vi "Autonomous Independent.vi"() -> ()   [LabVIEW 2018]
doc: "This VI is called when autonomous begins, and will automatically be terminated when autonomous ends. You can carry out timed or sensor driven robot movement independently without needing to return to the caller."
uses:
  <vilib>/Analysis/baseanly.llb/Mean (DBL).vi
  <vilib>/Rock Robotics/WPI/Utilities/WPI_GetSetVariantRefNum.vi
  <vilib>/Rock Robotics/Network Tables/NT Read Number.vi
  <vilib>/Rock Robotics/Network Tables/NT Write Numeric Array.vi
  <vilib>/Rock Robotics/Network Tables/NT Write String.vi
  Robot Global Data.vi
  <vilib>/Rock Robotics/WPI/RobotDrive/WPI_RobotDriveArcadeDrive_Standard(NoSaturation).vi
  <vilib>/Rock Robotics/Network Tables/NT Write Number.vi
  <vilib>/Analysis/NI_AALBase.lvlib
panel:
  in  "Array of robot movements":T1(array[cluster])=[{"X Joystick Value"=0.39393939393939403, "Y Joystick Value"=0.0, "Delay (sec)"=1.0, "Movement Name"="turn"}, {"X Joystick Value"=-0.3737373737373737, "Y Joystick Value"=0.0, "Delay (sec)"=1.0, "Movement Name"="turn back"}] {"Y Joystick Value" scale=1.0..-1.0; "X Joystick Value" scale=-1.0..1.0}
  out "Current Movement, for debugging":T2 {"Y Joystick Value" scale=1.0..-1.0; "X Joystick Value" scale=-1.0..1.0}
  # "Be sure to right-click and choose Data Operations>>Make Current Value default if you want to save the array values with the VI"
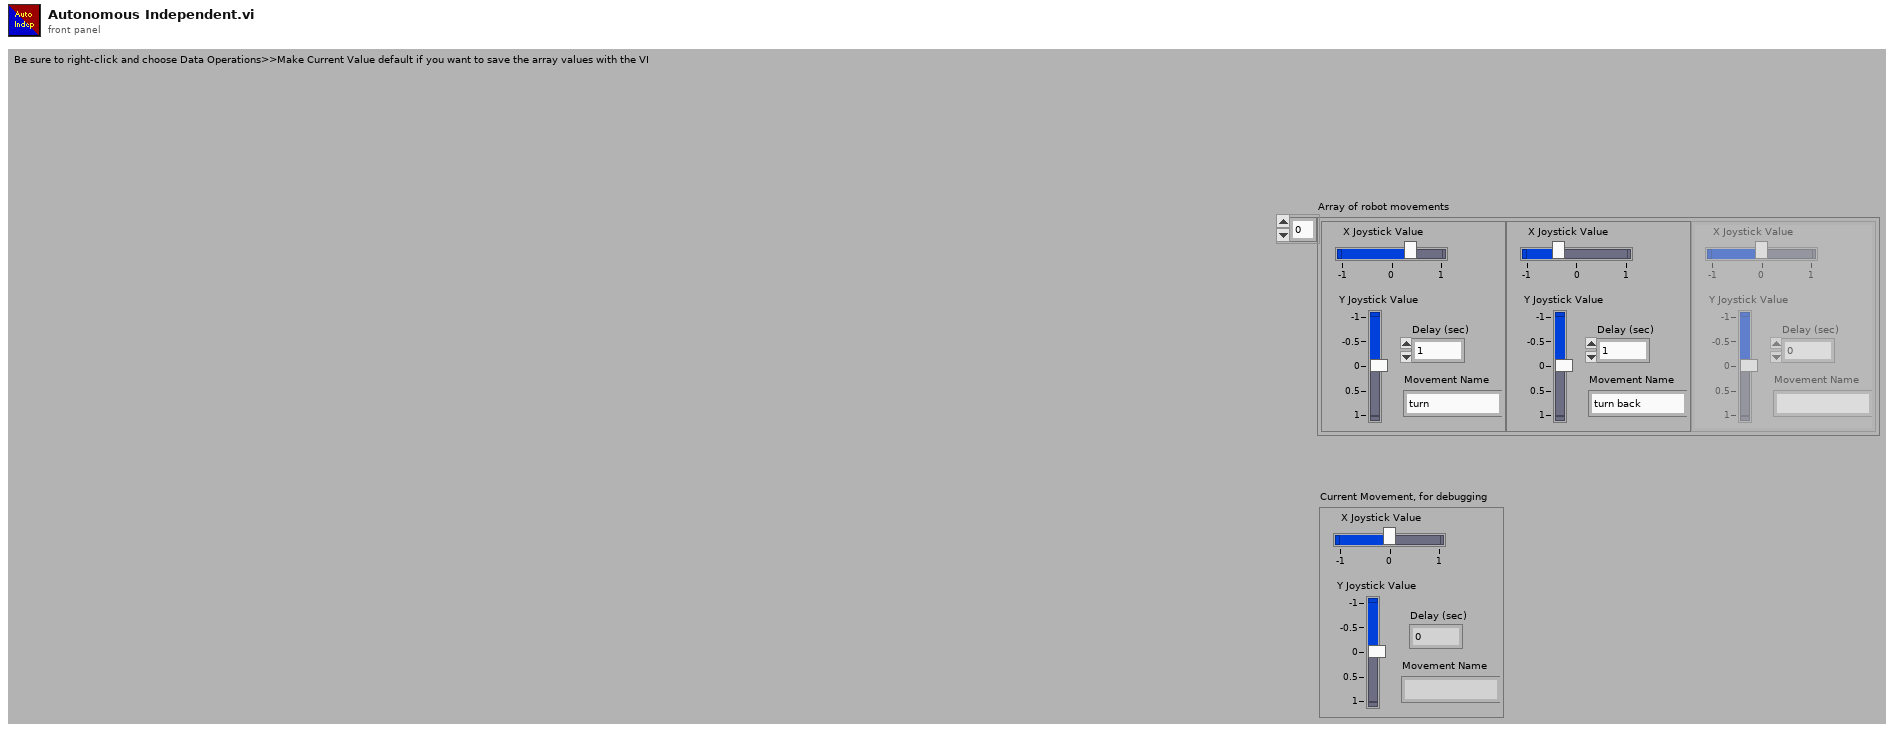
[diagram p1: front panel]
types:
  T1 = cluster{"X Joystick Value":dbl, "Y Joystick Value":dbl, "Delay (sec)":dbl, "Movement Name":string}[]
  T2 = cluster{"X Joystick Value":dbl, "Y Joystick Value":dbl, "Delay (sec)":dbl, "Movement Name":string}
  T3 = typedef "WPI_JoystickDevRef.ctl" = cluster{"Device":T4}
  T4 = typedef "WPI_JoystickDeviceEnum.ctl" = enum16{"USB 0", "USB 1", "USB 2", "USB 3", "USB 4", "USB 5"}
  T5 = typedef "WPI_RobotDriveDevRef.ctl" = cluster{"DevStatus":errorcluster, "Motors[]":T6[], "Square Inputs":bool, "Max Output":dbl}
  T6 = typedef "WPI_MotorControlDeviceRef.ctl" = cluster{"DeviceStatus":errorcluster, "Type":T7, "PWM":cluster{"PWM Channel":T8, "DeadBand":T9}, "CAN":cluster{"Device Number":u8, "SetOutput VI Ref":variant, "GetOutput VI Ref":variant, "Enable VI Ref":variant, "Disable VI Ref":variant, "Data":variant}, "Invert":bool, "DIO PWM":cluster{"PWM \"Enable\" Channel":T8, "DIOChannel":T10, "PWM Rate":dbl}}
  T7 = typedef "WPI_MotorControlType.ctl" = enum16{"PWM", "CAN", "DIO PWM"}
  T8 = typedef "FPGA_DIOPWMChannel.ctl" = enum8{"PWM 0", "PWM 1", "PWM 2", "PWM 3", "PWM 4", "PWM 5", "PWM 6", "PWM 7", "PWM 8", "PWM 9", "PWM MXP 0", "PWM MXP 1", "PWM MXP 2", "PWM MXP 3", "PWM MXP 4", "PWM MXP 5", "PWM MXP 6", "PWM MXP 7", "PWM MXP 8", "PWM MXP 9", "Invalid"}
  T9 = typedef "WPI_PWMDeadband.ctl" = cluster{"Name":string, "maxPositivePwm":i32, "minPositivePwm":i32, "centerPwm":i32, "maxNegativePwm":i32, "minNegativePwm":i32, "angularRange":u16}
  T10 = typedef "FPGA_DIOChannel.ctl" = enum8{"DIO 0", "DIO 1", "DIO 2", "DIO 3", "DIO 4", "DIO 5", "DIO 6", "DIO 7", "DIO 8", "DIO 9", "DIO MXP 0", "DIO MXP 1", "DIO MXP 2", "DIO MXP 3", "DIO MXP 4", "DIO MXP 5", "DIO MXP 6", "DIO MXP 7", "DIO MXP 8", "DIO MXP 9", "DIO MXP 10", "DIO MXP 11", "DIO MXP 12", "DIO MXP 13", "DIO MXP 14", "DIO MXP 15", "SPI Port CS1", "SPI Port CS2", "SPI Port CS3", "SPI Port MISO", "SPI Port MOSI", "Invalid"}
  T11 = typedef "WPI_AnalogChannelDevRef.ctl" = cluster{"DevStatus":errorcluster, "Analog Channel":T12}
  T12 = typedef "FPGA_AIChannel.ctl" = enum8{"AI 0", "AI 1", "AI 2", "AI 3", "AI MXP 0", "AI MXP 1", "AI MXP 2", "AI MXP 3", "Invalid"}
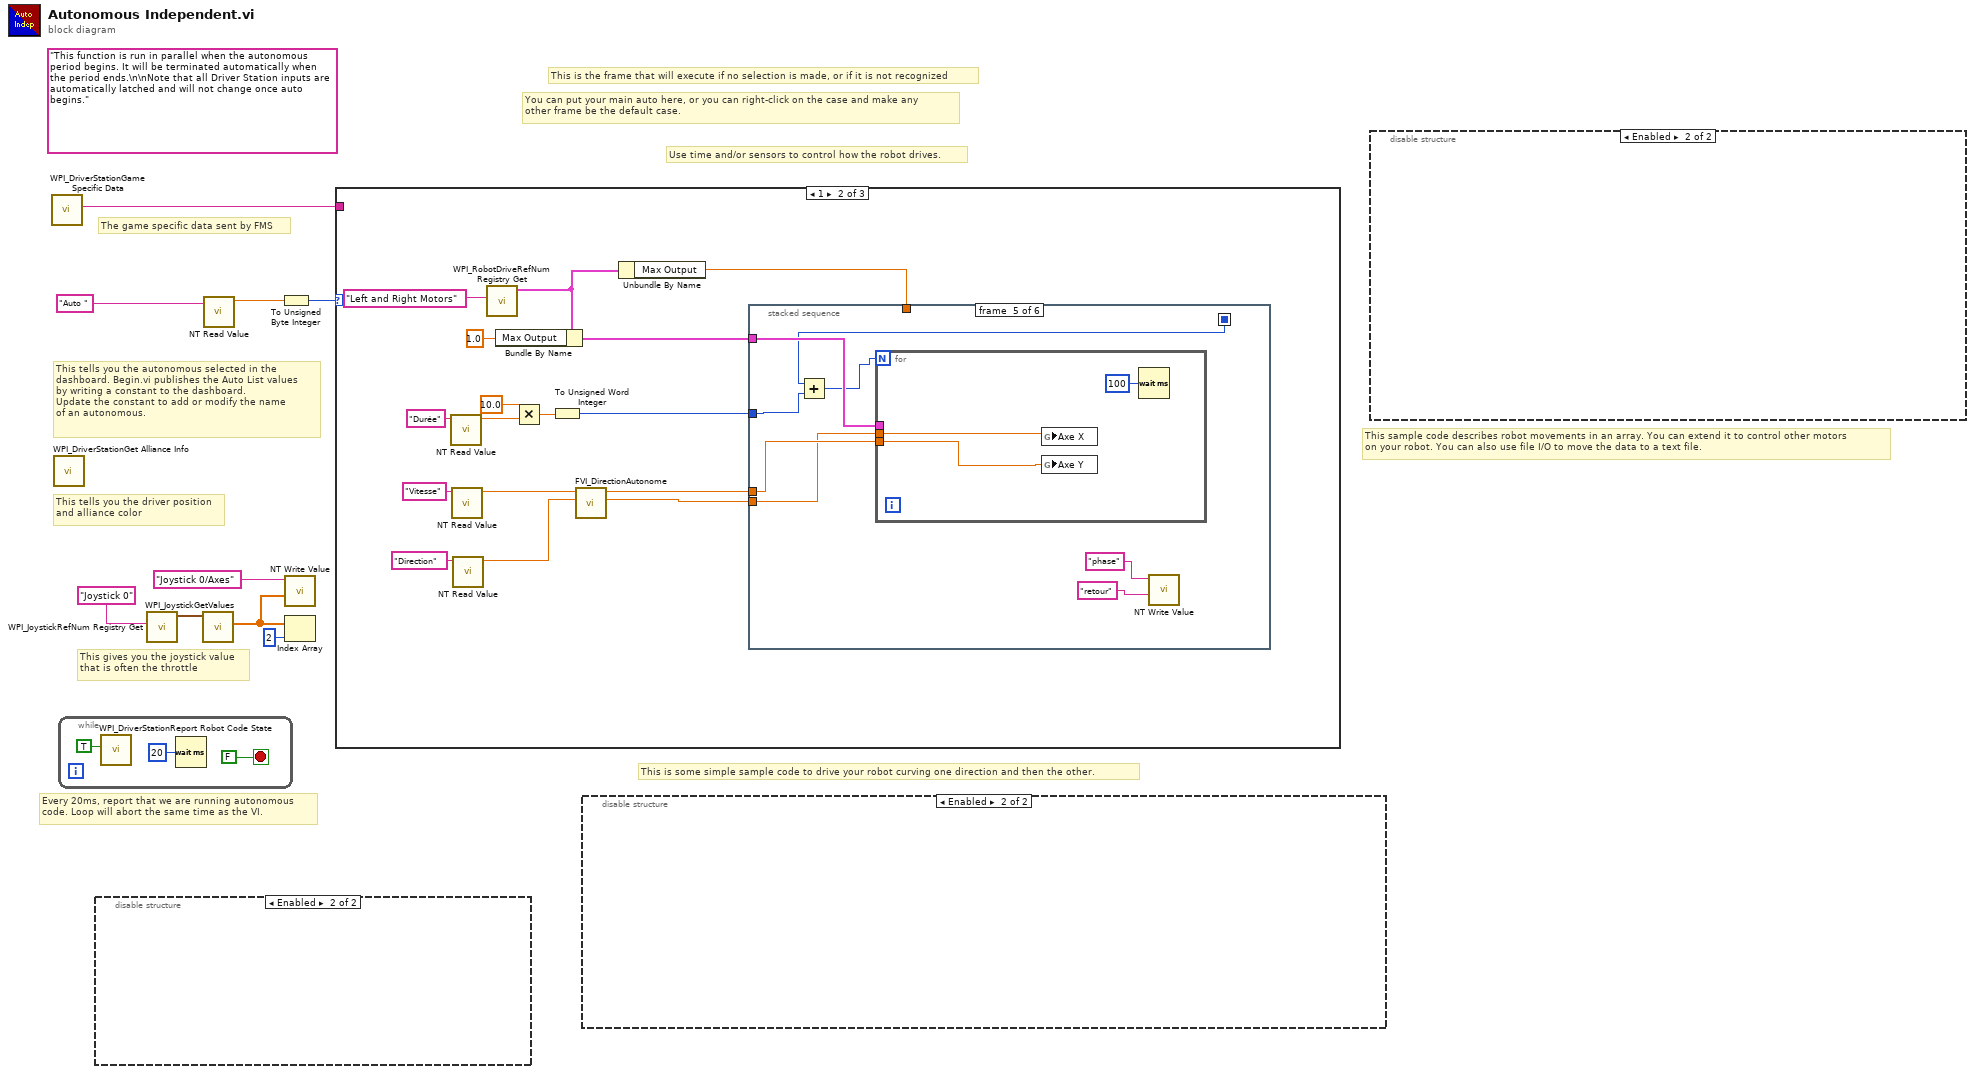
[diagram p0: block diagram]
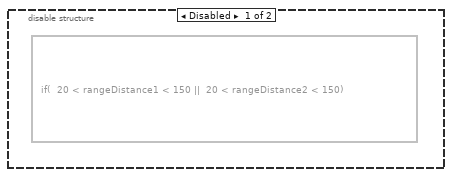
[diagram p2: hidden frame]
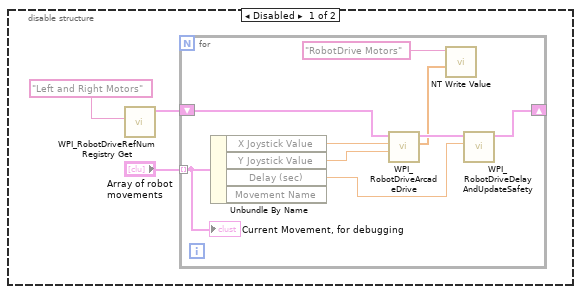
[diagram p3: hidden frame]
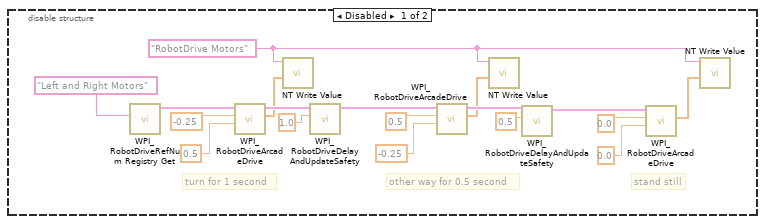
[diagram p4: hidden frame]
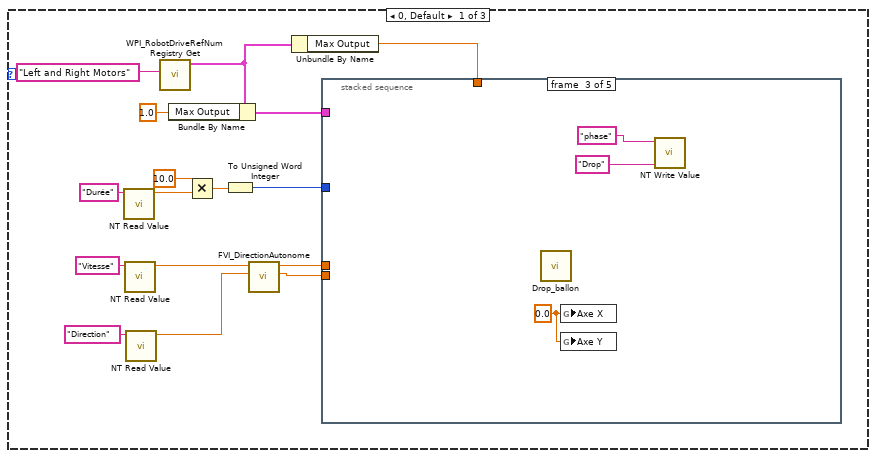
[diagram p5: hidden frame]
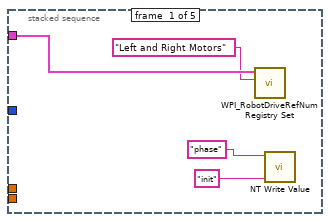
[diagram p6: hidden frame]
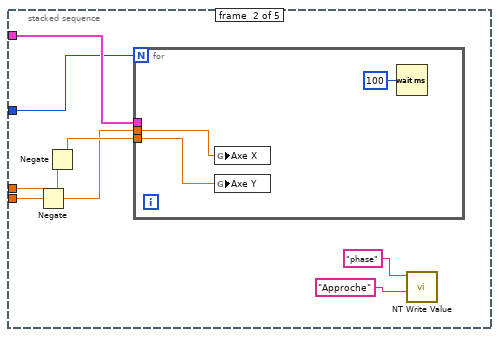
[diagram p7: hidden frame]
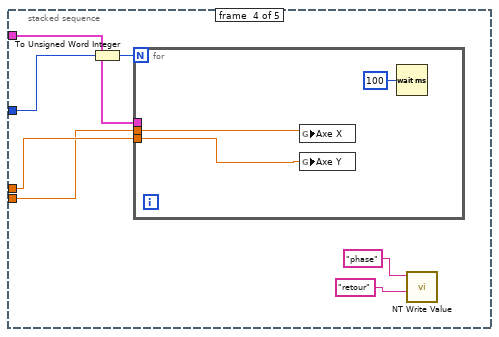
[diagram p8: hidden frame]
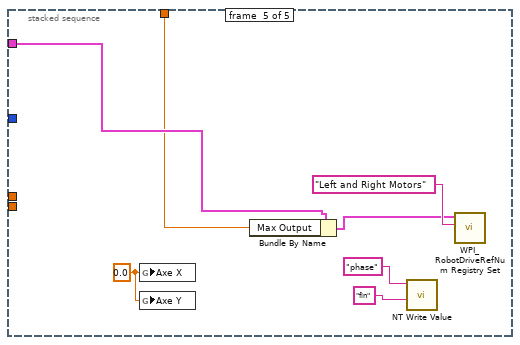
[diagram p9: hidden frame]
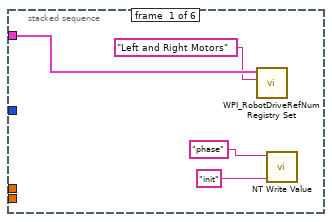
[diagram p10: hidden frame]
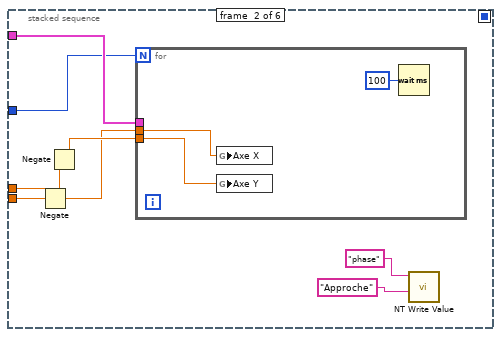
[diagram p11: hidden frame]
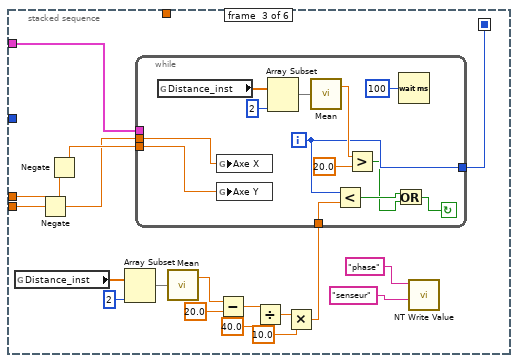
[diagram p12: hidden frame]
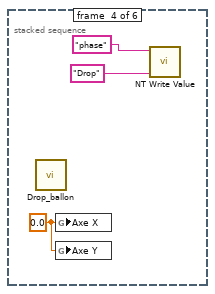
[diagram p13: hidden frame]
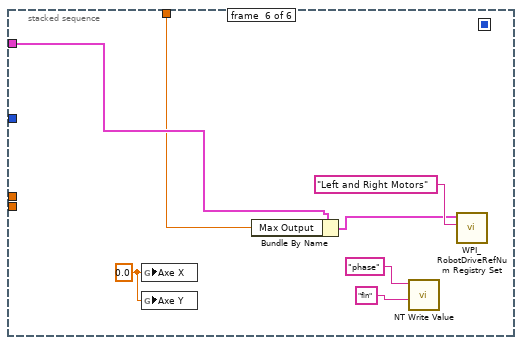
[diagram p14: hidden frame]
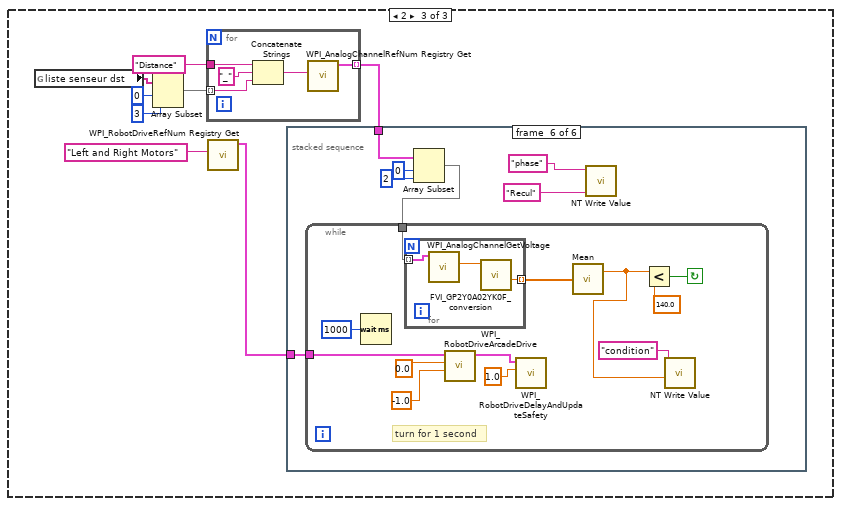
[diagram p15: hidden frame]
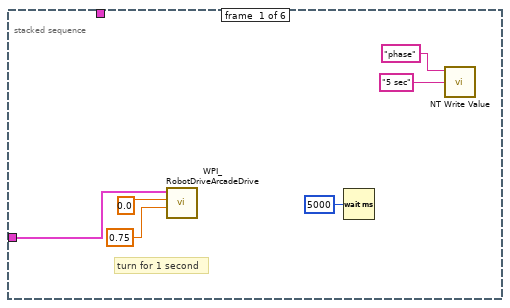
[diagram p16: hidden frame]
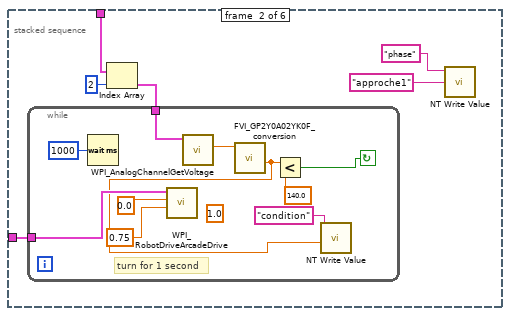
[diagram p17: hidden frame]
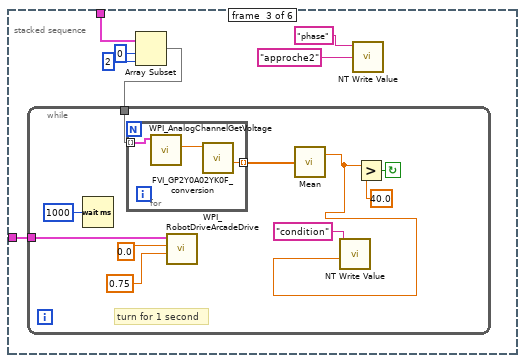
[diagram p18: hidden frame]
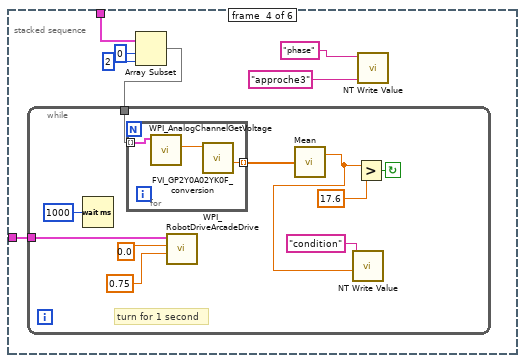
[diagram p19: hidden frame]
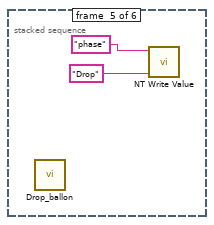
[diagram p20: hidden frame]
diagram:
  (unwired) "This function is run in parallel when the autonomous period begins. It will be terminated automatically when the period ends.\n\nNote that all Driver Station inputs are automatically latched and will not change once auto begins."
  # "You can put your main auto here, or you can right-click on the case and make any\nother frame be the default case."
  # "This is the frame that will execute if no selection is made, or if it is not recognized"
  # "This is some simple sample code to drive your robot curving one direction and then the other."
  # "This sample code describes robot movements in an array. You can extend it to control other motors\non your robot. You can also use file I/O to move the data to a text file."
  # "The game specific data sent by FMS"
  # "This tells you the autonomous selected in the \ndashboard. Begin.vi publishes the Auto List values\nby writing a constant to the dashboard.\nUpdate the constant to add or modify the name\nof an autonomous."
  # "Every 20ms, report that we are running autonomous\ncode. Loop will abort the same time as the VI."
  # "This gives you the joystick value\nthat is often the throttle"
  # "Use time and/or sensors to control how the robot drives."
  # "This tells you the driver position\nand alliance color"
  n1 = call <vilib>:"WPI_DriverStationGame Specific Data.vi"() -> ("Game Specific Data"=w2:string)  [unwired: 11 in]
  n2 = call <vilib>:"WPI_DriverStationGet Alliance Info.vi"() -> ()  [unwired: 12 out]
  n3 = while {
    stop <- FALSE stop-if-true
    n4 = call <vilib>:"WPI_DriverStationReport Robot Code State.vi"("Autonomous"=TRUE) -> ()  [unwired: 10 in, 1 out]
    n5 = Wait (ms)(milliseconds to wait=u32 20) -> ()  [unwired: 1 out]
  }
  n6 = disable-structure shown="Enabled" {
    frame Disabled {
      n7 = formula code="if(  20 < rangeDistance1 < 150 ||  20 < rangeDistance2 < 150)"() -> ()
    }
    frame Enabled {
    }
  }
  n8 = call <vilib>:"WPI_JoystickRefNum Registry Get.vi"("refnum name"="Joystick 0") -> ("JoystickDevRef"=w8:T3)  [unwired: 1 in, 9 out]
  n9 = call <vilib>:"WPI_JoystickGetValues.vi"("JoystickDevRef"=w8) -> ("Axes"=w4:dbl[])  [unwired: 6 in, 4 out]
  n10 = call-poly <vilib>:"NT Read Value.vi"("Name"="Auto ") -> ("Numeric"=w5:dbl)  [unwired: 9 in, 1 out]
  n11 = To Unsigned Byte Integer(number=w5) -> (unsigned 8bit integer=w1:u8)
  n12 = call-poly <vilib>:"NT Write Value.vi"("Numeric Array"=w4, "Name"="Joystick 0/Axes") -> ()  [unwired: 9 in, 1 out]
  n13 = Index Array(array=w4, index=2) -> ()  [unwired: 1 out]
  n14 = case shown="1" w1 {
    tunnel: w2 -> [_ _ _]
    frame 0, Default {
      n15 = call-poly <vilib>:"NT Read Value.vi"("Name"="Durée") -> ("Numeric"=w24:dbl)  [unwired: 9 in, 1 out]
      n16 = call-poly <vilib>:"NT Read Value.vi"("Name"="Vitesse") -> ("Numeric"=w20:dbl)  [unwired: 9 in, 1 out]
      n17 = call-poly <vilib>:"NT Read Value.vi"("Name"="Direction") -> ("Numeric"=w19:dbl)  [unwired: 9 in, 1 out]
      n18 = call <vilib>:"WPI_RobotDriveRefNum Registry Get.vi"("refnum name"="Left and Right Motors") -> ("RobotDriveDevRef"=w15:T5)  [unwired: 1 in, 9 out]
      n19 = Bundle By Name(cluster=w15, "Max Output"=1.0) -> (w14:T5)
      n20 = Multiply(x=10.0, y=w24) -> (x*y=w22:dbl)
      n21 = To Unsigned Word Integer(number=w22) -> (unsigned 16bit integer=w21:u16)
      n22 = call "FVI_DirectionAutonome.vi"("Direction"=w19, "vitesse"=w20) -> ("x"=w17:dbl, "y"=w18:dbl)  [unwired: 8 in]
      n23 = Unbundle By Name(w15) -> ("Max Output"=w13:dbl)
      n24 = stacked-sequence {
        tunnel: w14 -> [w32 w40 _ w53 w60]
        tunnel: w21 -> [_ w39 _ w47 _]
        tunnel: w18 -> [_ w38 _ w52 _]
        tunnel: w17 -> [_ w37 _ w51 _]
        tunnel: w13 -> [_ _ _ _ w57]
        frame #0 {
          n25 = call <vilib>:"WPI_RobotDriveRefNum Registry Set.vi"("refnum name"="Left and Right Motors", "RobotDriveDevRef"=w32) -> ()  [unwired: 8 in, 2 out]
          n26 = call-poly <vilib>:"NT Write Value.vi"("String"="init", "Name"="phase") -> ()  [unwired: 9 in, 1 out]
        }
        frame #1 {
          n27 = Negate(x=w37) -> (-x=w33:dbl)
          n28 = Negate(x=w38) -> (-x=w34:dbl)
          n29 = for {
            N: w39 -> [_]
            tunnel: w40 -> [_]
            tunnel: w34 -> [w41]
            tunnel: w33 -> [w42]
            n30 = global write "Robot Global Data.vi" "Axe X"(w42) -> ()
            n31 = global write "Robot Global Data.vi" "Axe Y"(w41) -> ()
            n32 = Wait (ms)(milliseconds to wait=u32 100) -> ()  [unwired: 1 out]
          }
          n33 = call-poly <vilib>:"NT Write Value.vi"("String"="Approche", "Name"="phase") -> ()  [unwired: 9 in, 1 out]
        }
        frame #2 {
          w44 = 0.0 ("Axe X")
          n34 = call "Drop_ballon.vi"() -> ()  [unwired: 12 in]
          n35 = global write "Robot Global Data.vi" "Axe X"(w44) -> ()
          n36 = global write "Robot Global Data.vi" "Axe Y"(w44) -> ()
          n37 = call-poly <vilib>:"NT Write Value.vi"("String"="Drop", "Name"="phase") -> ()  [unwired: 9 in, 1 out]
        }
        frame #3 {
          n38 = To Unsigned Word Integer(number=w47) -> (unsigned 16bit integer=w48:u16)
          n39 = for {
            N: w48 -> [_]
            tunnel: w53 -> [_]
            tunnel: w52 -> [w54]
            tunnel: w51 -> [w55]
            n40 = global write "Robot Global Data.vi" "Axe X"(w55) -> ()
            n41 = global write "Robot Global Data.vi" "Axe Y"(w54) -> ()
            n42 = Wait (ms)(milliseconds to wait=u32 100) -> ()  [unwired: 1 out]
          }
          n43 = call-poly <vilib>:"NT Write Value.vi"("String"="retour", "Name"="phase") -> ()  [unwired: 9 in, 1 out]
        }
        frame #4 {
          w58 = 0.0 ("Axe X")
          n44 = global write "Robot Global Data.vi" "Axe X"(w58) -> ()
          n45 = global write "Robot Global Data.vi" "Axe Y"(w58) -> ()
          n46 = Bundle By Name(cluster=w60, "Max Output"=w57) -> (w59:T5)
          n47 = call-poly <vilib>:"NT Write Value.vi"("String"="fin", "Name"="phase") -> ()  [unwired: 9 in, 1 out]
          n48 = call <vilib>:"WPI_RobotDriveRefNum Registry Set.vi"("refnum name"="Left and Right Motors", "RobotDriveDevRef"=w59) -> ()  [unwired: 8 in, 2 out]
        }
      }
    }
    frame 1 {
      n49 = call-poly <vilib>:"NT Read Value.vi"("Name"="Durée") -> ("Numeric"=w75:dbl)  [unwired: 9 in, 1 out]
      n50 = call-poly <vilib>:"NT Read Value.vi"("Name"="Vitesse") -> ("Numeric"=w71:dbl)  [unwired: 9 in, 1 out]
      n51 = call-poly <vilib>:"NT Read Value.vi"("Name"="Direction") -> ("Numeric"=w70:dbl)  [unwired: 9 in, 1 out]
      n52 = call <vilib>:"WPI_RobotDriveRefNum Registry Get.vi"("refnum name"="Left and Right Motors") -> ("RobotDriveDevRef"=w66:T5)  [unwired: 1 in, 9 out]
      n53 = Bundle By Name(cluster=w66, "Max Output"=1.0) -> (w65:T5)
      n54 = Multiply(x=10.0, y=w75) -> (x*y=w73:dbl)
      n55 = To Unsigned Word Integer(number=w73) -> (unsigned 16bit integer=w72:u16)
      n56 = call "FVI_DirectionAutonome.vi"("Direction"=w70, "vitesse"=w71) -> ("x"=w68:dbl, "y"=w69:dbl)  [unwired: 8 in]
      n57 = Unbundle By Name(w66) -> ("Max Output"=w64:dbl)
      n58 = stacked-sequence {
        seq-local: [_ _ w105 _ _ _] -> [_ _ _ _ w130 _]
        tunnel: w65 -> [w83 w91 w112 _ w136 w143]
        tunnel: w72 -> [_ w90 _ _ w131 _]
        tunnel: w69 -> [_ w89 w111 _ w135 _]
        tunnel: w68 -> [_ w88 w110 _ w134 _]
        tunnel: w64 -> [_ _ _ _ _ w140]
        frame #0 {
          n59 = call <vilib>:"WPI_RobotDriveRefNum Registry Set.vi"("refnum name"="Left and Right Motors", "RobotDriveDevRef"=w83) -> ()  [unwired: 8 in, 2 out]
          n60 = call-poly <vilib>:"NT Write Value.vi"("String"="init", "Name"="phase") -> ()  [unwired: 9 in, 1 out]
        }
        frame #1 {
          n61 = Negate(x=w88) -> (-x=w84:dbl)
          n62 = Negate(x=w89) -> (-x=w85:dbl)
          n63 = for {
            N: w90 -> [_]
            tunnel: w91 -> [_]
            tunnel: w85 -> [w92]
            tunnel: w84 -> [w93]
            n64 = global write "Robot Global Data.vi" "Axe X"(w93) -> ()
            n65 = global write "Robot Global Data.vi" "Axe Y"(w92) -> ()
            n66 = Wait (ms)(milliseconds to wait=u32 100) -> ()  [unwired: 1 out]
          }
          n67 = call-poly <vilib>:"NT Write Value.vi"("String"="Approche", "Name"="phase") -> ()  [unwired: 9 in, 1 out]
        }
        frame #2 {
          n68 = global read "Robot Global Data.vi" "Distance_inst"() -> (w102:dbl[])
          n69 = Negate(x=w110) -> (-x=w106:dbl)
          n70 = Negate(x=w111) -> (-x=w107:dbl)
          n71 = Array Subset(array=w102, length=2) -> (w104:dbl[])  [unwired: 1 in]
          n72 = call-poly <vilib>:"Mean.vi"("X"=w104) -> ("mean"=w101:dbl)  [unwired: 1 out]
          n73 = Subtract(x=w101, y=20.0) -> (x-y=w99:dbl)
          n74 = Divide(x=w99, y=40.0) -> (x/y=w97:dbl)
          n75 = Multiply(x=w97, y=10.0) -> (x*y=w95:dbl)
          n76 = while {
            tunnel: w112 -> [_]
            tunnel: w107 -> [w123]
            tunnel: w106 -> [w124]
            tunnel: [w117] -> w105
            tunnel: w95 -> [w116]
            i -> [w117]
            stop <- w113 continue-if-true
            n77 = global read "Robot Global Data.vi" "Distance_inst"() -> (w122:dbl[])
            n78 = global write "Robot Global Data.vi" "Axe X"(w124) -> ()
            n79 = global write "Robot Global Data.vi" "Axe Y"(w123) -> ()
            n80 = Array Subset(array=w122, length=2) -> (w120:dbl[])  [unwired: 1 in]
            n81 = call-poly <vilib>:"Mean.vi"("X"=w120) -> ("mean"=w119:dbl)  [unwired: 1 out]
            n82 = Less?(x=w117, y=w116) -> (x < y?=w115:bool)
            n83 = Greater?(x=w119, y=20.0) -> (0:w114:bool)
            n84 = Or(x=w115, y=w114) -> (x .or. y?=w113:bool)
            n85 = Wait (ms)(milliseconds to wait=u32 100) -> ()  [unwired: 1 out]
          }
          n86 = call-poly <vilib>:"NT Write Value.vi"("String"="senseur", "Name"="phase") -> ()  [unwired: 9 in, 1 out]
        }
        frame #3 {
          w126 = 0.0 ("Axe X")
          n87 = call "Drop_ballon.vi"() -> ()  [unwired: 12 in]
          n88 = global write "Robot Global Data.vi" "Axe X"(w126) -> ()
          n89 = global write "Robot Global Data.vi" "Axe Y"(w126) -> ()
          n90 = call-poly <vilib>:"NT Write Value.vi"("String"="Drop", "Name"="phase") -> ()  [unwired: 9 in, 1 out]
        }
        frame #4 {
          n91 = Add(x=w130, y=w131) -> (x+y=w129:i32)
          n92 = for {
            N: w129 -> [_]
            tunnel: w136 -> [_]
            tunnel: w135 -> [w137]
            tunnel: w134 -> [w138]
            n93 = global write "Robot Global Data.vi" "Axe X"(w138) -> ()
            n94 = global write "Robot Global Data.vi" "Axe Y"(w137) -> ()
            n95 = Wait (ms)(milliseconds to wait=u32 100) -> ()  [unwired: 1 out]
          }
          n96 = call-poly <vilib>:"NT Write Value.vi"("String"="retour", "Name"="phase") -> ()  [unwired: 9 in, 1 out]
        }
        frame #5 {
          w141 = 0.0 ("Axe X")
          n97 = global write "Robot Global Data.vi" "Axe X"(w141) -> ()
          n98 = global write "Robot Global Data.vi" "Axe Y"(w141) -> ()
          n99 = Bundle By Name(cluster=w143, "Max Output"=w140) -> (w142:T5)
          n100 = call-poly <vilib>:"NT Write Value.vi"("String"="fin", "Name"="phase") -> ()  [unwired: 9 in, 1 out]
          n101 = call <vilib>:"WPI_RobotDriveRefNum Registry Set.vi"("refnum name"="Left and Right Motors", "RobotDriveDevRef"=w142) -> ()  [unwired: 8 in, 2 out]
        }
      }
    }
    frame 2 {
      n102 = global read "Robot Global Data.vi" "liste senseur dst"() -> (w151:string[])
      n103 = Array Subset(array=w151, index=0, length=3) -> (w152:string[])
      n104 = for {
        tunnel: "Distance" -> [w245]
        tunnel: w152 -> [w243] mode=indexing
        tunnel: [w241] -> w147 mode=indexing
        n105 = Concatenate Strings(w245, "_" ("string"), w243) -> (w242:string)
        n106 = call <vilib>:"WPI_AnalogChannelRefNum Registry Get.vi"("refnum name"=w242) -> ("AIDeviceRef"=w241:T11)  [unwired: 9 in, 1 out]
      }
      n107 = call <vilib>:"WPI_RobotDriveRefNum Registry Get.vi"("refnum name"="Left and Right Motors") -> ("RobotDriveDevRef"=w153:T5)  [unwired: 1 in, 9 out]
      n108 = stacked-sequence {
        tunnel: w153 -> [w160 w166 w183 w203 _ w225]
        tunnel: w147 -> [_ w165 w182 w202 _ w224]
        frame #0 {
          # "turn for 1 second"
          n109 = call-poly <vilib>:"WPI_RobotDriveArcadeDrive.vi"("Y axis value"=0.75 ("X axis value"), "X axis value"=0.0, "RobotDriveDevRef"=w160) -> ()  [unwired: 1 in, 8 out]
          n110 = Wait (ms)(milliseconds to wait=u32 5000) -> ()  [unwired: 1 out]
          n111 = call-poly <vilib>:"NT Write Value.vi"("String"="5 sec", "Name"="phase") -> ()  [unwired: 9 in, 1 out]
        }
        frame #1 {
          n112 = Index Array(array=w165, index=2) -> (element=w163:T11)
          n113 = while {
            tunnel: w166 -> [w173]
            tunnel: w163 -> [w171]
            stop <- w169 continue-if-true
            (unwired) 1.0 ("Delay (s)")
            # "turn for 1 second"
            n114 = Wait (ms)(milliseconds to wait=u32 1000) -> ()  [unwired: 1 out]
            n115 = call-poly <vilib>:"WPI_RobotDriveArcadeDrive.vi"("Y axis value"=0.75 ("X axis value"), "X axis value"=0.0, "RobotDriveDevRef"=w173) -> ()  [unwired: 1 in, 8 out]
            n116 = call <vilib>:"WPI_AnalogChannelGetVoltage.vi"("AIDeviceRef"=w171) -> ("Voltage"=w172:dbl)  [unwired: 8 in, 2 out]
            n117 = call "FVI_GP2Y0A02YK0F_conversion.vi"("Voltage"=w172) -> ("x-y"=w167:dbl)  [unwired: 10 in]
            n118 = Less?(x=w167, y=140.0) -> (x < y?=w169:bool)
            n119 = call-poly <vilib>:"NT Write Value.vi"("Numeric"=w167, "Name"="condition") -> ()  [unwired: 9 in, 1 out]
          }
          n120 = call-poly <vilib>:"NT Write Value.vi"("String"="approche1", "Name"="phase") -> ()  [unwired: 9 in, 1 out]
        }
        frame #2 {
          n121 = Array Subset(array=w182, index=0, length=2) -> (w179:T11[])
          n122 = while {
            tunnel: w183 -> [w190]
            tunnel: w179 -> [w187]
            stop <- w188 continue-if-true
            # "turn for 1 second"
            n123 = Wait (ms)(milliseconds to wait=u32 1000) -> ()  [unwired: 1 out]
            n124 = for {
              tunnel: w187 -> [w195] mode=indexing
              tunnel: [w194] -> w186 mode=indexing
              n125 = call <vilib>:"WPI_AnalogChannelGetVoltage.vi"("AIDeviceRef"=w195) -> ("Voltage"=w196:dbl)  [unwired: 8 in, 2 out]
              n126 = call "FVI_GP2Y0A02YK0F_conversion.vi"("Voltage"=w196) -> ("x-y"=w194:dbl)  [unwired: 10 in]
            }
            n127 = call-poly <vilib>:"WPI_RobotDriveArcadeDrive.vi"("Y axis value"=0.75 ("X axis value"), "X axis value"=0.0, "RobotDriveDevRef"=w190) -> ()  [unwired: 1 in, 8 out]
            n128 = call-poly <vilib>:"Mean.vi"("X"=w186) -> ("mean"=w184:dbl)  [unwired: 1 out]
            n129 = call-poly <vilib>:"NT Write Value.vi"("Numeric"=w184, "Name"="condition") -> ()  [unwired: 9 in, 1 out]
            n130 = Greater?(x=w184, y=40.0) -> (0:w188:bool)
          }
          n131 = call-poly <vilib>:"NT Write Value.vi"("String"="approche2", "Name"="phase") -> ()  [unwired: 9 in, 1 out]
        }
        frame #3 {
          n132 = Array Subset(array=w202, index=0, length=2) -> (w199:T11[])
          n133 = while {
            tunnel: w203 -> [w210]
            tunnel: w199 -> [w207]
            stop <- w208 continue-if-true
            # "turn for 1 second"
            n134 = Wait (ms)(milliseconds to wait=u32 1000) -> ()  [unwired: 1 out]
            n135 = for {
              tunnel: w207 -> [w215] mode=indexing
              tunnel: [w214] -> w206 mode=indexing
              n136 = call <vilib>:"WPI_AnalogChannelGetVoltage.vi"("AIDeviceRef"=w215) -> ("Voltage"=w216:dbl)  [unwired: 8 in, 2 out]
              n137 = call "FVI_GP2Y0A02YK0F_conversion.vi"("Voltage"=w216) -> ("x-y"=w214:dbl)  [unwired: 10 in]
            }
            n138 = call-poly <vilib>:"WPI_RobotDriveArcadeDrive.vi"("Y axis value"=0.75 ("X axis value"), "X axis value"=0.0, "RobotDriveDevRef"=w210) -> ()  [unwired: 1 in, 8 out]
            n139 = call-poly <vilib>:"Mean.vi"("X"=w206) -> ("mean"=w204:dbl)  [unwired: 1 out]
            n140 = call-poly <vilib>:"NT Write Value.vi"("Numeric"=w204, "Name"="condition") -> ()  [unwired: 9 in, 1 out]
            n141 = Greater?(x=w204, y=17.6) -> (0:w208:bool)
          }
          n142 = call-poly <vilib>:"NT Write Value.vi"("String"="approche3", "Name"="phase") -> ()  [unwired: 9 in, 1 out]
        }
        frame #4 {
          n143 = call "Drop_ballon.vi"() -> ()  [unwired: 12 in]
          n144 = call-poly <vilib>:"NT Write Value.vi"("String"="Drop", "Name"="phase") -> ()  [unwired: 9 in, 1 out]
        }
        frame #5 {
          n145 = Array Subset(array=w224, index=0, length=2) -> (w221:T11[])
          n146 = while {
            tunnel: w225 -> [w232]
            tunnel: w221 -> [w231]
            stop <- w228 continue-if-true
            # "turn for 1 second"
            n147 = Wait (ms)(milliseconds to wait=u32 1000) -> ()  [unwired: 1 out]
            n148 = for {
              tunnel: w231 -> [w239] mode=indexing
              tunnel: [w238] -> w230 mode=indexing
              n149 = call <vilib>:"WPI_AnalogChannelGetVoltage.vi"("AIDeviceRef"=w239) -> ("Voltage"=w240:dbl)  [unwired: 8 in, 2 out]
              n150 = call "FVI_GP2Y0A02YK0F_conversion.vi"("Voltage"=w240) -> ("x-y"=w238:dbl)  [unwired: 10 in]
            }
            n151 = call-poly <vilib>:"WPI_RobotDriveArcadeDrive.vi"("Y axis value"=-1.0 ("X axis value"), "X axis value"=0.0, "RobotDriveDevRef"=w232) -> ("RobotDriveDevRef"=w234:T5)  [unwired: 1 in, 7 out]
            n152 = call <vilib>:"WPI_RobotDriveDelayAndUpdateSafety.vi"("Delay (s)"=1.0, "RobotDriveDevRef"=w234) -> ()  [unwired: 8 in, 2 out]
            n153 = call-poly <vilib>:"Mean.vi"("X"=w230) -> ("mean"=w226:dbl)  [unwired: 1 out]
            n154 = Less?(x=w226, y=140.0) -> (x < y?=w228:bool)
            n155 = call-poly <vilib>:"NT Write Value.vi"("Numeric"=w226, "Name"="condition") -> ()  [unwired: 9 in, 1 out]
          }
          n156 = call-poly <vilib>:"NT Write Value.vi"("String"="Recul", "Name"="phase") -> ()  [unwired: 9 in, 1 out]
        }
      }
    }
  }
  n157 = disable-structure shown="Enabled" {
    frame Disabled {
      w247 = "RobotDrive Motors" ("Name")
      # "stand still"
      # "other way for 0.5 second"
      # "turn for 1 second"
      n158 = call <vilib>:"WPI_RobotDriveRefNum Registry Get.vi"("refnum name"="Left and Right Motors") -> ("RobotDriveDevRef"=w263:T5)  [unwired: 1 in, 9 out]
      n159 = call-poly <vilib>:"WPI_RobotDriveArcadeDrive.vi"("Y axis value"=0.5 ("X axis value"), "X axis value"=-0.25, "RobotDriveDevRef"=w263) -> ("Motor Values"=w246:dbl[], "RobotDriveDevRef"=w256:T5)  [unwired: 1 in, 6 out]
      n160 = call-poly <vilib>:"NT Write Value.vi"("Numeric Array"=w246, "Name"=w247) -> ()  [unwired: 9 in, 1 out]
      n161 = call <vilib>:"WPI_RobotDriveDelayAndUpdateSafety.vi"("Delay (s)"=1.0, "RobotDriveDevRef"=w256) -> ("RobotDriveDevRef 2"=w257:T5)  [unwired: 8 in, 1 out]
      n162 = call-poly <vilib>:"WPI_RobotDriveArcadeDrive.vi"("Y axis value"=-0.25 ("X axis value"), "X axis value"=0.5, "RobotDriveDevRef"=w257) -> ("Motor Values"=w248:dbl[], "RobotDriveDevRef"=w258:T5)  [unwired: 1 in, 6 out]
      n163 = call-poly <vilib>:"NT Write Value.vi"("Numeric Array"=w248, "Name"=w247) -> ()  [unwired: 9 in, 1 out]
      n164 = call <vilib>:"WPI_RobotDriveDelayAndUpdateSafety.vi"("Delay (s)"=0.5, "RobotDriveDevRef"=w258) -> ("RobotDriveDevRef 2"=w259:T5)  [unwired: 8 in, 1 out]
      n165 = call-poly <vilib>:"WPI_RobotDriveArcadeDrive.vi"("Y axis value"=0.0 ("X axis value"), "X axis value"=0.0, "RobotDriveDevRef"=w259) -> ("Motor Values"=w249:dbl[])  [unwired: 1 in, 7 out]
      n166 = call-poly <vilib>:"NT Write Value.vi"("Numeric Array"=w249, "Name"=w247) -> ()  [unwired: 9 in, 1 out]
    }
    frame Enabled {
    }
  }
  n167 = disable-structure shown="Enabled" {
    frame Disabled {
      n168 = call <vilib>:"WPI_RobotDriveRefNum Registry Get.vi"("refnum name"="Left and Right Motors") -> ("RobotDriveDevRef"=w265:T5)  [unwired: 1 in, 9 out]
      n169 = for {
        shift-right: [w273] -> _
        shift-left: w265 -> [w274]
        tunnel: "Array of robot movements" -> [w269] mode=indexing
        n170 = Unbundle By Name(w269) -> ("X Joystick Value"=w272:dbl, "Y Joystick Value"=w271:dbl, "Delay (sec)"=w270:dbl)  [unwired: 1 out]
        n171 = call-poly <vilib>:"WPI_RobotDriveArcadeDrive.vi"("Y axis value"=w271, "X axis value"=w272, "RobotDriveDevRef"=w274) -> ("Motor Values"=w267:dbl[], "RobotDriveDevRef"=w275:T5)  [unwired: 1 in, 6 out]
        n172 = call-poly <vilib>:"NT Write Value.vi"("Numeric Array"=w267, "Name"="RobotDrive Motors") -> ()  [unwired: 9 in, 1 out]
        n173 = call <vilib>:"WPI_RobotDriveDelayAndUpdateSafety.vi"("Delay (s)"=w270, "RobotDriveDevRef"=w275) -> ("RobotDriveDevRef 2"=w273:T5)  [unwired: 8 in, 1 out]
        "Current Movement, for debugging" <- w269
      }
    }
    frame Enabled {
    }
  }
